vi "String Label-Value Replacement.vi"(3 "token array":string[](array[string])=["value1"], 4 "index array":i32[](array[numeric])=[1], 5 "string in":string="ChargingState=CHARGE_OFF-0\r\nChargeWarning=NO\r\nTemperatureLevel=1\r\nIPG_ReceivedLevel=1") -> (2 "string out":string)   [LabVIEW 2010]
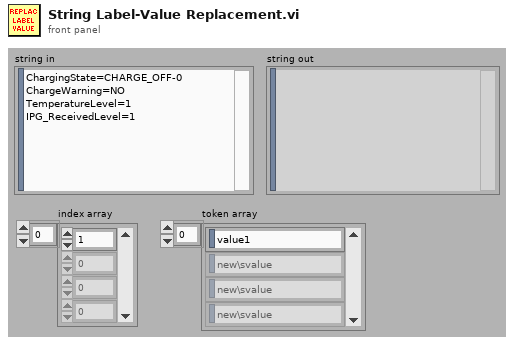
[diagram p1: front panel]
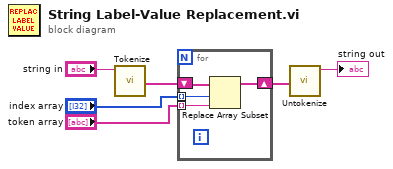
[diagram p0: block diagram]
diagram:
  n1 = call "Tokenize.vi"("input string"="string in") -> ("tokens"=w4:string[])  [unwired: 4 in, 2 out]
  n2 = for {
    shift-right: [w10] -> w3
    shift-left: w4 -> [w9]
    tunnel: "index array" -> [w8] mode=indexing
    tunnel: "token array" -> [w7] mode=indexing
    n3 = Replace Array Subset(array=w9, new element=w7, index=w8) -> (w10:string[])
  }
  n4 = call "Untokenize.vi"("tokens"=w3) -> ("string out"=→"string out":string)  [unwired: 10 in]
